vi "check noise source.vi"(8 "PLC bool write Tags":T1={"AT set glass wand lower"={"Tag Name"="S060.PXI.Signals.PlltData.SN", "Network Path"="172.15.51.1,1,0", "use opc"=FALSE, "DataSocket Reference"={"CWDSLib._DCWDataSocket"=refnum, "CWDSLib._DCWData"=refnum, "OnDataUpdated"=0, "OnStatusUpdated"=0}}, "AT set sunshade wand lower"={"Tag Name"="S060.PXI.Signals.PlltData.SN", "Network Path"="172.15.51.1,1,0", "use opc"=FALSE, "DataSocket Reference"={"CWDSLib._DCWDataSocket"=refnum, "CWDSLib._DCWData"=refnum, "OnDataUpdated"=0, "OnStatusUpdated"=0}}, "AT set sunshade wand up"={"Tag Name"="S060.PXI.Signals.PlltData.SN", "Network Path"="172.15.51.1,1,0", "use opc"=FALSE, "DataSocket Reference"={"CWDSLib._DCWDataSocket"=refnum, "CWDSLib._DCWData"=refnum, "OnDataUpdated"=0, "OnStatusUpdated"=0}}, "AT set glass wand up"={"Tag Name"="S060.PXI.Signals.PlltData.SN", "Network Path"="172.15.51.1,1,0", "use opc"=FALSE, "DataSocket Reference"={"CWDSLib._DCWDataSocket"=refnum, "CWDSLib._DCWData"=refnum, "OnDataUpdated"=0, "OnStatusUpdated"=0}}, "AT set wand home pos"={"Tag Name"="S060.PXI.Signals.PlltData.SN", "Network Path"="172.15.51.1,1,0", "use opc"=FALSE, "DataSocket Reference"={"CWDSLib._DCWDataSocket"=refnum, "CWDSLib._DCWData"=refnum, "OnDataUpdated"=0, "OnStatusUpdated"=0}}, "Test Complete Pass"={"Tag Name"="S060.PXI.Signals.PlltData.SN", "Network Path"="172.15.51.1,1,0", "use opc"=FALSE, "DataSocket Reference"={"CWDSLib._DCWDataSocket"=refnum, "CWDSLib._DCWData"=refnum, "OnDataUpdated"=0, "OnStatusUpdated"=0}}, "Test Complete Fail"={"Tag Name"="S060.PXI.Signals.PlltData.SN", "Network Path"="172.15.51.1,1,0", "use opc"=FALSE, "DataSocket Reference"={"CWDSLib._DCWDataSocket"=refnum, "CWDSLib._DCWData"=refnum, "OnDataUpdated"=0, "OnStatusUpdated"=0}}, "Test Started"={"Tag Name"="S060.PXI.Signals.PlltData.SN", "Network Path"="172.15.51.1,1,0", "use opc"=FALSE, "DataSocket Reference"={"CWDSLib._DCWDataSocket"=refnum, "CWDSLib._DCWData"=refnum, "OnDataUpdated"=0, "OnStatusUpdated"=0}}, "Retract LVDT's"={"Tag Name"="S060.PXI.Signals.PlltData.SN", "Network Path"="172.15.51.1,1,0", "use opc"=FALSE, "DataSocket Reference"={"CWDSLib._DCWDataSocket"=refnum, "CWDSLib._DCWData"=refnum, "OnDataUpdated"=0, "OnStatusUpdated"=0}}, "Extend LVDT's"={"Tag Name"="S060.PXI.Signals.PlltData.SN", "Network Path"="172.15.51.1,1,0", "use opc"=FALSE, "DataSocket Reference"={"CWDSLib._DCWDataSocket"=refnum, "CWDSLib._DCWData"=refnum, "OnDataUpdated"=0, "OnStatusUpdated"=0}}, "ss servo open"={"Tag Name"="S060.PXI.Signals.PlltData.SN", "Network Path"="172.15.51.1,1,0", "use opc"=FALSE, "DataSocket Reference"={"CWDSLib._DCWDataSocket"=refnum, "CWDSLib._DCWData"=refnum, "OnDataUpdated"=0, "OnStatusUpdated"=0}}, "ss servo close"={"Tag Name"="S060.PXI.Signals.PlltData.SN", "Network Path"="172.15.51.1,1,0", "use opc"=FALSE, "DataSocket Reference"={"CWDSLib._DCWDataSocket"=refnum, "CWDSLib._DCWData"=refnum, "OnDataUpdated"=0, "OnStatusUpdated"=0}}, "control slide start"={"Tag Name"="S060.PXI.Signals.PlltData.SN", "Network Path"="172.15.51.1,1,0", "use opc"=FALSE, "DataSocket Reference"={"CWDSLib._DCWDataSocket"=refnum, "CWDSLib._DCWData"=refnum, "OnDataUpdated"=0, "OnStatusUpdated"=0}}, "control slide stop"={"Tag Name"="S060.PXI.Signals.PlltData.SN", "Network Path"="172.15.51.1,1,0", "use opc"=FALSE, "DataSocket Reference"={"CWDSLib._DCWDataSocket"=refnum, "CWDSLib._DCWData"=refnum, "OnDataUpdated"=0, "OnStatusUpdated"=0}}, "AT VentPMACHome"={"Tag Name"="S060.PXI.Signals.PlltData.SN", "Network Path"="172.15.51.1,1,0", "use opc"=FALSE, "DataSocket Reference"={"CWDSLib._DCWDataSocket"=refnum, "CWDSLib._DCWData"=refnum, "OnDataUpdated"=0, "OnStatusUpdated"=0}}, "AT VentPMACExtended"={"Tag Name"="S060.PXI.Signals.PlltData.SN", "Network Path"="172.15.51.1,1,0", "use opc"=FALSE, "DataSocket Reference"={"CWDSLib._DCWDataSocket"=refnum, "CWDSLib._DCWData"=refnum, "OnDataUpdated"=0, "OnStatusUpdated"=0}}, "Good Frame Barcode"={"Tag Name"="S060.PXI.Signals.PlltData.SN", "Network Path"="172.15.51.1,1,0", "use opc"=FALSE, "DataSocket Reference"={"CWDSLib._DCWDataSocket"=refnum, "CWDSLib._DCWData"=refnum, "OnDataUpdated"=0, "OnStatusUpdated"=0}}, "Bad Frame Barcode"={"Tag Name"="S060.PXI.Signals.PlltData.SN", "Network Path"="172.15.51.1,1,0", "use opc"=FALSE, "DataSocket Reference"={"CWDSLib._DCWDataSocket"=refnum, "CWDSLib._DCWData"=refnum, "OnDataUpdated"=0, "OnStatusUpdated"=0}}, "Extend Z LVDTS"={"Tag Name"="S060.PXI.Signals.PlltData.SN", "Network Path"="172.15.51.1,1,0", "use opc"=FALSE, "DataSocket Reference"={"CWDSLib._DCWDataSocket"=refnum, "CWDSLib._DCWData"=refnum, "OnDataUpdated"=0, "OnStatusUpdated"=0}}, "NVH SunRoof Moving"={"Tag Name"="S060.PXI.Signals.PlltData.SN", "Network Path"="172.15.51.1,1,0", "use opc"=FALSE, "DataSocket Reference"={"CWDSLib._DCWDataSocket"=refnum, "CWDSLib._DCWData"=refnum, "OnDataUpdated"=0, "OnStatusUpdated"=0}}, "NVH SunRoof Stop"={"Tag Name"="S060.PXI.Signals.PlltData.SN", "Network Path"="172.15.51.1,1,0", "use opc"=FALSE, "DataSocket Reference"={"CWDSLib._DCWDataSocket"=refnum, "CWDSLib._DCWData"=refnum, "OnDataUpdated"=0, "OnStatusUpdated"=0}}, "NVH Pass"={"Tag Name"="S060.PXI.Signals.PlltData.SN", "Network Path"="172.15.51.1,1,0", "use opc"=FALSE, "DataSocket Reference"={"CWDSLib._DCWDataSocket"=refnum, "CWDSLib._DCWData"=refnum, "OnDataUpdated"=0, "OnStatusUpdated"=0}}, "NVH Fail"={"Tag Name"="S060.PXI.Signals.PlltData.SN", "Network Path"="172.15.51.1,1,0", "use opc"=FALSE, "DataSocket Reference"={"CWDSLib._DCWDataSocket"=refnum, "CWDSLib._DCWData"=refnum, "OnDataUpdated"=0, "OnStatusUpdated"=0}}, "NVH Operator Express Glass Opened"={"Tag Name"="S060.PXI.Signals.PlltData.SN", "Network Path"="172.15.51.1,1,0", "use opc"=FALSE, "DataSocket Reference"={"CWDSLib._DCWDataSocket"=refnum, "CWDSLib._DCWData"=refnum, "OnDataUpdated"=0, "OnStatusUpdated"=0}}, "NVH Operator Express Glass Closed"={"Tag Name"="S060.PXI.Signals.PlltData.SN", "Network Path"="172.15.51.1,1,0", "use opc"=FALSE, "DataSocket Reference"={"CWDSLib._DCWDataSocket"=refnum, "CWDSLib._DCWData"=refnum, "OnDataUpdated"=0, "OnStatusUpdated"=0}}, "NVH Operator Express Rollo Opened01"={"Tag Name"="S060.PXI.Signals.PlltData.SN", "Network Path"="172.15.51.1,1,0", "use opc"=FALSE, "DataSocket Reference"={"CWDSLib._DCWDataSocket"=refnum, "CWDSLib._DCWData"=refnum, "OnDataUpdated"=0, "OnStatusUpdated"=0}}, "NVH Operator Express Rollo Closed01"={"Tag Name"="S060.PXI.Signals.PlltData.SN", "Network Path"="172.15.51.1,1,0", "use opc"=FALSE, "DataSocket Reference"={"CWDSLib._DCWDataSocket"=refnum, "CWDSLib._DCWData"=refnum, "OnDataUpdated"=0, "OnStatusUpdated"=0}}, "NVH Operator Express Rollo Opened02"={"Tag Name"="S060.PXI.Signals.PlltData.SN", "Network Path"="172.15.51.1,1,0", "use opc"=FALSE, "DataSocket Reference"={"CWDSLib._DCWDataSocket"=refnum, "CWDSLib._DCWData"=refnum, "OnDataUpdated"=0, "OnStatusUpdated"=0}}, "NVH Operator Pass"={"Tag Name"="S060.PXI.Signals.PlltData.SN", "Network Path"="172.15.51.1,1,0", "use opc"=FALSE, "DataSocket Reference"={"CWDSLib._DCWDataSocket"=refnum, "CWDSLib._DCWData"=refnum, "OnDataUpdated"=0, "OnStatusUpdated"=0}}, "NVH Operator Fail"={"Tag Name"="S060.PXI.Signals.PlltData.SN", "Network Path"="172.15.51.1,1,0", "use opc"=FALSE, "DataSocket Reference"={"CWDSLib._DCWDataSocket"=refnum, "CWDSLib._DCWData"=refnum, "OnDataUpdated"=0, "OnStatusUpdated"=0}}, "NVH Operator Check"={"Tag Name"="S060.PXI.Signals.PlltData.SN", "Network Path"="172.15.51.1,1,0", "use opc"=FALSE, "DataSocket Reference"={"CWDSLib._DCWDataSocket"=refnum, "CWDSLib._DCWData"=refnum, "OnDataUpdated"=0, "OnStatusUpdated"=0}}, "NVH Operator Vent Open Noise"={"Tag Name"="S060.PXI.Signals.PlltData.SN", "Network Path"="172.15.51.1,1,0", "use opc"=FALSE, "DataSocket Reference"={"CWDSLib._DCWDataSocket"=refnum, "CWDSLib._DCWData"=refnum, "OnDataUpdated"=0, "OnStatusUpdated"=0}}, "NVH Operator Vent Close Noise"={"Tag Name"="S060.PXI.Signals.PlltData.SN", "Network Path"="172.15.51.1,1,0", "use opc"=FALSE, "DataSocket Reference"={"CWDSLib._DCWDataSocket"=refnum, "CWDSLib._DCWData"=refnum, "OnDataUpdated"=0, "OnStatusUpdated"=0}}, "NVH Operator Sunshade Open Noise"={"Tag Name"="S060.PXI.Signals.PlltData.SN", "Network Path"="172.15.51.1,1,0", "use opc"=FALSE, "DataSocket Reference"={"CWDSLib._DCWDataSocket"=refnum, "CWDSLib._DCWData"=refnum, "OnDataUpdated"=0, "OnStatusUpdated"=0}}, "NVH Operator Sunshade Close Noise"={"Tag Name"="S060.PXI.Signals.PlltData.SN", "Network Path"="172.15.51.1,1,0", "use opc"=FALSE, "DataSocket Reference"={"CWDSLib._DCWDataSocket"=refnum, "CWDSLib._DCWData"=refnum, "OnDataUpdated"=0, "OnStatusUpdated"=0}}, "NVH Operator Glass Open Noise"={"Tag Name"="S060.PXI.Signals.PlltData.SN", "Network Path"="172.15.51.1,1,0", "use opc"=FALSE, "DataSocket Reference"={"CWDSLib._DCWDataSocket"=refnum, "CWDSLib._DCWData"=refnum, "OnDataUpdated"=0, "OnStatusUpdated"=0}}, "NVH Operator Glass Close Noise"={"Tag Name"="S060.PXI.Signals.PlltData.SN", "Network Path"="172.15.51.1,1,0", "use opc"=FALSE, "DataSocket Reference"={"CWDSLib._DCWDataSocket"=refnum, "CWDSLib._DCWData"=refnum, "OnDataUpdated"=0, "OnStatusUpdated"=0}}, "NVH Operator Finish"={"Tag Name"="S060.PXI.Signals.PlltData.SN", "Network Path"="172.15.51.1,1,0", "use opc"=FALSE, "DataSocket Reference"={"CWDSLib._DCWDataSocket"=refnum, "CWDSLib._DCWData"=refnum, "OnDataUpdated"=0, "OnStatusUpdated"=0}}, "Barcode01 OK"={"Tag Name"="S060.PXI.Signals.PlltData.SN", "Network Path"="172.15.51.1,1,0", "use opc"=FALSE, "DataSocket Reference"={"CWDSLib._DCWDataSocket"=refnum, "CWDSLib._DCWData"=refnum, "OnDataUpdated"=0, "OnStatusUpdated"=0}}, "Barcode02 OK"={"Tag Name"="S060.PXI.Signals.PlltData.SN", "Network Path"="172.15.51.1,1,0", "use opc"=FALSE, "DataSocket Reference"={"CWDSLib._DCWDataSocket"=refnum, "CWDSLib._DCWData"=refnum, "OnDataUpdated"=0, "OnStatusUpdated"=0}}, "AT set to Vent ATS Test Pos"={"Tag Name"="S060.PXI.Signals.PlltData.SN", "Network Path"="172.15.51.1,1,0", "use opc"=FALSE, "DataSocket Reference"={"CWDSLib._DCWDataSocket"=refnum, "CWDSLib._DCWData"=refnum, "OnDataUpdated"=0, "OnStatusUpdated"=0}}, "AT set to Vent ATS Home Pos"={"Tag Name"="S060.PXI.Signals.PlltData.SN", "Network Path"="172.15.51.1,1,0", "use opc"=FALSE, "DataSocket Reference"={"CWDSLib._DCWDataSocket"=refnum, "CWDSLib._DCWData"=refnum, "OnDataUpdated"=0, "OnStatusUpdated"=0}}, "Move LVDT Adjust Station"={"Tag Name"="S060.PXI.Signals.PlltData.SN", "Network Path"="172.15.51.1,1,0", "use opc"=FALSE, "DataSocket Reference"={"CWDSLib._DCWDataSocket"=refnum, "CWDSLib._DCWData"=refnum, "OnDataUpdated"=0, "OnStatusUpdated"=0}}} {"Move LVDT Adjust Station"."DataSocket Reference"."OnStatusUpdated" format="%.0x"; "Move LVDT Adjust Station"."DataSocket Reference"."OnDataUpdated" format="%.0x"; "AT set to Vent ATS Home Pos"."DataSocket Reference"."OnStatusUpdated" format="%.0x"; "AT set to Vent ATS Home Pos"."DataSocket Reference"."OnDataUpdated" format="%.0x"; "AT set to Vent ATS Test Pos"."DataSocket Reference"."OnStatusUpdated" format="%.0x"; "AT set to Vent ATS Test Pos"."DataSocket Reference"."OnDataUpdated" format="%.0x"; "Barcode02 OK"."DataSocket Reference"."OnStatusUpdated" format="%.0x"; "Barcode02 OK"."DataSocket Reference"."OnDataUpdated" format="%.0x"; "Barcode01 OK"."DataSocket Reference"."OnStatusUpdated" format="%.0x"; "Barcode01 OK"."DataSocket Reference"."OnDataUpdated" format="%.0x"; "AT set glass wand up"."DataSocket Reference"."OnStatusUpdated" format="%.0x"; "AT set glass wand up"."DataSocket Reference"."OnDataUpdated" format="%.0x"; "AT set sunshade wand up"."DataSocket Reference"."OnStatusUpdated" format="%.0x"; "AT set sunshade wand up"."DataSocket Reference"."OnDataUpdated" format="%.0x"; "NVH Operator Finish"."DataSocket Reference"."OnStatusUpdated" format="%.0x"; "NVH Operator Finish"."DataSocket Reference"."OnDataUpdated" format="%.0x"; "NVH Operator Glass Close Noise"."DataSocket Reference"."OnStatusUpdated" format="%.0x"; "NVH Operator Glass Close Noise"."DataSocket Reference"."OnDataUpdated" format="%.0x"; "NVH Operator Glass Open Noise"."DataSocket Reference"."OnStatusUpdated" format="%.0x"; "NVH Operator Glass Open Noise"."DataSocket Reference"."OnDataUpdated" format="%.0x"; "NVH Operator Sunshade Close Noise"."DataSocket Reference"."OnStatusUpdated" format="%.0x"; "NVH Operator Sunshade Close Noise"."DataSocket Reference"."OnDataUpdated" format="%.0x"; "NVH Operator Sunshade Open Noise"."DataSocket Reference"."OnStatusUpdated" format="%.0x"; "NVH Operator Sunshade Open Noise"."DataSocket Reference"."OnDataUpdated" format="%.0x"; "NVH Operator Vent Close Noise"."DataSocket Reference"."OnStatusUpdated" format="%.0x"; "NVH Operator Vent Close Noise"."DataSocket Reference"."OnDataUpdated" format="%.0x"; "NVH Operator Vent Open Noise"."DataSocket Reference"."OnStatusUpdated" format="%.0x"; "NVH Operator Vent Open Noise"."DataSocket Reference"."OnDataUpdated" format="%.0x"; "NVH Operator Check"."DataSocket Reference"."OnStatusUpdated" format="%.0x"; "NVH Operator Check"."DataSocket Reference"."OnDataUpdated" format="%.0x"; "NVH Operator Fail"."DataSocket Reference"."OnStatusUpdated" format="%.0x"; "NVH Operator Fail"."DataSocket Reference"."OnDataUpdated" format="%.0x"; "NVH Operator Pass"."DataSocket Reference"."OnStatusUpdated" format="%.0x"; "NVH Operator Pass"."DataSocket Reference"."OnDataUpdated" format="%.0x"; "NVH Operator Express Rollo Opened02"."DataSocket Reference"."OnStatusUpdated" format="%.0x"; "NVH Operator Express Rollo Opened02"."DataSocket Reference"."OnDataUpdated" format="%.0x"; "NVH Operator Express Rollo Closed01"."DataSocket Reference"."OnStatusUpdated" format="%.0x"; "NVH Operator Express Rollo Closed01"."DataSocket Reference"."OnDataUpdated" format="%.0x"; "NVH Operator Express Rollo Opened01"."DataSocket Reference"."OnStatusUpdated" format="%.0x"; "NVH Operator Express Rollo Opened01"."DataSocket Reference"."OnDataUpdated" format="%.0x"; "NVH Operator Express Glass Closed"."DataSocket Reference"."OnStatusUpdated" format="%.0x"; "NVH Operator Express Glass Closed"."DataSocket Reference"."OnDataUpdated" format="%.0x"; "NVH Operator Express Glass Opened"."DataSocket Reference"."OnStatusUpdated" format="%.0x"; "NVH Operator Express Glass Opened"."DataSocket Reference"."OnDataUpdated" format="%.0x"; "NVH Fail"."DataSocket Reference"."OnStatusUpdated" format="%.0x"; "NVH Fail"."DataSocket Reference"."OnDataUpdated" format="%.0x"; "NVH Pass"."DataSocket Reference"."OnStatusUpdated" format="%.0x"; "NVH Pass"."DataSocket Reference"."OnDataUpdated" format="%.0x"; "NVH SunRoof Stop"."DataSocket Reference"."OnStatusUpdated" format="%.0x"; "NVH SunRoof Stop"."DataSocket Reference"."OnDataUpdated" format="%.0x"; "NVH SunRoof Moving"."DataSocket Reference"."OnStatusUpdated" format="%.0x"; "NVH SunRoof Moving"."DataSocket Reference"."OnDataUpdated" format="%.0x"; "Extend Z LVDTS"."DataSocket Reference"."OnStatusUpdated" format="%.0x"; "Extend Z LVDTS"."DataSocket Reference"."OnDataUpdated" format="%.0x"; "Bad Frame Barcode"."DataSocket Reference"."OnStatusUpdated" format="%.0x"; "Bad Frame Barcode"."DataSocket Reference"."OnDataUpdated" format="%.0x"; "Good Frame Barcode"."DataSocket Reference"."OnStatusUpdated" format="%.0x"; "Good Frame Barcode"."DataSocket Reference"."OnDataUpdated" format="%.0x"; "AT VentPMACExtended"."DataSocket Reference"."OnStatusUpdated" format="%.0x"; "AT VentPMACExtended"."DataSocket Reference"."OnDataUpdated" format="%.0x"; "AT VentPMACHome"."DataSocket Reference"."OnStatusUpdated" format="%.0x"; "AT VentPMACHome"."DataSocket Reference"."OnDataUpdated" format="%.0x"; "control slide stop"."DataSocket Reference"."OnStatusUpdated" format="%.0x"; "control slide stop"."DataSocket Reference"."OnDataUpdated" format="%.0x"; "control slide start"."DataSocket Reference"."OnStatusUpdated" format="%.0x"; "control slide start"."DataSocket Reference"."OnDataUpdated" format="%.0x"; "ss servo close"."DataSocket Reference"."OnStatusUpdated" format="%.0x"; "ss servo close"."DataSocket Reference"."OnDataUpdated" format="%.0x"; "ss servo open"."DataSocket Reference"."OnStatusUpdated" format="%.0x"; "ss servo open"."DataSocket Reference"."OnDataUpdated" format="%.0x"; "Extend LVDT's"."DataSocket Reference"."OnStatusUpdated" format="%.0x"; "Extend LVDT's"."DataSocket Reference"."OnDataUpdated" format="%.0x"; "Retract LVDT's"."DataSocket Reference"."OnStatusUpdated" format="%.0x"; "Retract LVDT's"."DataSocket Reference"."OnDataUpdated" format="%.0x"; "Test Started"."DataSocket Reference"."OnStatusUpdated" format="%.0x"; "Test Started"."DataSocket Reference"."OnDataUpdated" format="%.0x"; "Test Complete Fail"."DataSocket Reference"."OnStatusUpdated" format="%.0x"; "Test Complete Fail"."DataSocket Reference"."OnDataUpdated" format="%.0x"; "Test Complete Pass"."DataSocket Reference"."OnStatusUpdated" format="%.0x"; "Test Complete Pass"."DataSocket Reference"."OnDataUpdated" format="%.0x"; "AT set wand home pos"."DataSocket Reference"."OnStatusUpdated" format="%.0x"; "AT set wand home pos"."DataSocket Reference"."OnDataUpdated" format="%.0x"; "AT set sunshade wand lower"."DataSocket Reference"."OnStatusUpdated" format="%.0x"; "AT set sunshade wand lower"."DataSocket Reference"."OnDataUpdated" format="%.0x"; "AT set glass wand lower"."DataSocket Reference"."OnStatusUpdated" format="%.0x"; "AT set glass wand lower"."DataSocket Reference"."OnDataUpdated" format="%.0x"}, 9 "Noise Source Input":u32, 10 "Error Table In":string[][](table), 11 "input cluster":T4={"AT glass position"={"Tag Name"="S060.PXI.Signals.PlltData.SN", "Network Path"="172.15.51.1,1,0", "use opc"=FALSE, "DataSocket Reference"={"CWDSLib._DCWDataSocket"=refnum, "CWDSLib._DCWData"=refnum, "OnDataUpdated"=0, "OnStatusUpdated"=0}}, "AT shade position"={"Tag Name"="S060.PXI.Signals.PlltData.SN", "Network Path"="172.15.51.1,1,0", "use opc"=FALSE, "DataSocket Reference"={"CWDSLib._DCWDataSocket"=refnum, "CWDSLib._DCWData"=refnum, "OnDataUpdated"=0, "OnStatusUpdated"=0}}, "AT in glass wand lower pos"={"Tag Name"="S060.PXI.Signals.PlltData.SN", "Network Path"="172.15.51.1,1,0", "use opc"=FALSE, "DataSocket Reference"={"CWDSLib._DCWDataSocket"=refnum, "CWDSLib._DCWData"=refnum, "OnDataUpdated"=0, "OnStatusUpdated"=0}}, "AT in glass wand up pos"={"Tag Name"="S060.PXI.Signals.PlltData.SN", "Network Path"="172.15.51.1,1,0", "use opc"=FALSE, "DataSocket Reference"={"CWDSLib._DCWDataSocket"=refnum, "CWDSLib._DCWData"=refnum, "OnDataUpdated"=0, "OnStatusUpdated"=0}}, "AT in sunshad wand lower pos"={"Tag Name"="S060.PXI.Signals.PlltData.SN", "Network Path"="172.15.51.1,1,0", "use opc"=FALSE, "DataSocket Reference"={"CWDSLib._DCWDataSocket"=refnum, "CWDSLib._DCWData"=refnum, "OnDataUpdated"=0, "OnStatusUpdated"=0}}, "AT in sunshad wand up pos"={"Tag Name"="S060.PXI.Signals.PlltData.SN", "Network Path"="172.15.51.1,1,0", "use opc"=FALSE, "DataSocket Reference"={"CWDSLib._DCWDataSocket"=refnum, "CWDSLib._DCWData"=refnum, "OnDataUpdated"=0, "OnStatusUpdated"=0}}, "AT in wand home pos"={"Tag Name"="S060.PXI.Signals.PlltData.SN", "Network Path"="172.15.51.1,1,0", "use opc"=FALSE, "DataSocket Reference"={"CWDSLib._DCWDataSocket"=refnum, "CWDSLib._DCWData"=refnum, "OnDataUpdated"=0, "OnStatusUpdated"=0}}, "LVDT's Extended"={"Tag Name"="S060.PXI.Signals.PlltData.SN", "Network Path"="172.15.51.1,1,0", "use opc"=FALSE, "DataSocket Reference"={"CWDSLib._DCWDataSocket"=refnum, "CWDSLib._DCWData"=refnum, "OnDataUpdated"=0, "OnStatusUpdated"=0}}, "bolt check 1"={"Tag Name"="S060.PXI.Signals.PlltData.SN", "Network Path"="172.15.51.1,1,0", "use opc"=FALSE, "DataSocket Reference"={"CWDSLib._DCWDataSocket"=refnum, "CWDSLib._DCWData"=refnum, "OnDataUpdated"=0, "OnStatusUpdated"=0}}, "bolt check 2"={"Tag Name"="S060.PXI.Signals.PlltData.SN", "Network Path"="172.15.51.1,1,0", "use opc"=FALSE, "DataSocket Reference"={"CWDSLib._DCWDataSocket"=refnum, "CWDSLib._DCWData"=refnum, "OnDataUpdated"=0, "OnStatusUpdated"=0}}, "bolt check 3"={"Tag Name"="S060.PXI.Signals.PlltData.SN", "Network Path"="172.15.51.1,1,0", "use opc"=FALSE, "DataSocket Reference"={"CWDSLib._DCWDataSocket"=refnum, "CWDSLib._DCWData"=refnum, "OnDataUpdated"=0, "OnStatusUpdated"=0}}, "bolt check 4"={"Tag Name"="S060.PXI.Signals.PlltData.SN", "Network Path"="172.15.51.1,1,0", "use opc"=FALSE, "DataSocket Reference"={"CWDSLib._DCWDataSocket"=refnum, "CWDSLib._DCWData"=refnum, "OnDataUpdated"=0, "OnStatusUpdated"=0}}, "bolt check 5"={"Tag Name"="S060.PXI.Signals.PlltData.SN", "Network Path"="172.15.51.1,1,0", "use opc"=FALSE, "DataSocket Reference"={"CWDSLib._DCWDataSocket"=refnum, "CWDSLib._DCWData"=refnum, "OnDataUpdated"=0, "OnStatusUpdated"=0}}, "bolt check 6"={"Tag Name"="S060.PXI.Signals.PlltData.SN", "Network Path"="172.15.51.1,1,0", "use opc"=FALSE, "DataSocket Reference"={"CWDSLib._DCWDataSocket"=refnum, "CWDSLib._DCWData"=refnum, "OnDataUpdated"=0, "OnStatusUpdated"=0}}, "bolt check 7"={"Tag Name"="S060.PXI.Signals.PlltData.SN", "Network Path"="172.15.51.1,1,0", "use opc"=FALSE, "DataSocket Reference"={"CWDSLib._DCWDataSocket"=refnum, "CWDSLib._DCWData"=refnum, "OnDataUpdated"=0, "OnStatusUpdated"=0}}, "bolt check 8"={"Tag Name"="S060.PXI.Signals.PlltData.SN", "Network Path"="172.15.51.1,1,0", "use opc"=FALSE, "DataSocket Reference"={"CWDSLib._DCWDataSocket"=refnum, "CWDSLib._DCWData"=refnum, "OnDataUpdated"=0, "OnStatusUpdated"=0}}, "start"={"Tag Name"="S060.PXI.Signals.PlltData.SN", "Network Path"="172.15.51.1,1,0", "use opc"=FALSE, "DataSocket Reference"={"CWDSLib._DCWDataSocket"=refnum, "CWDSLib._DCWData"=refnum, "OnDataUpdated"=0, "OnStatusUpdated"=0}}, "abort"={"Tag Name"="S060.PXI.Signals.PlltData.SN", "Network Path"="172.15.51.1,1,0", "use opc"=FALSE, "DataSocket Reference"={"CWDSLib._DCWDataSocket"=refnum, "CWDSLib._DCWData"=refnum, "OnDataUpdated"=0, "OnStatusUpdated"=0}}, "LVDT's Retracted"={"Tag Name"="S060.PXI.Signals.PlltData.SN", "Network Path"="172.15.51.1,1,0", "use opc"=FALSE, "DataSocket Reference"={"CWDSLib._DCWDataSocket"=refnum, "CWDSLib._DCWData"=refnum, "OnDataUpdated"=0, "OnStatusUpdated"=0}}, "manual barcode print"={"Tag Name"="S060.PXI.Signals.PlltData.SN", "Network Path"="172.15.51.1,1,0", "use opc"=FALSE, "DataSocket Reference"={"CWDSLib._DCWDataSocket"=refnum, "CWDSLib._DCWData"=refnum, "OnDataUpdated"=0, "OnStatusUpdated"=0}}, "ss servo at open"={"Tag Name"="S060.PXI.Signals.PlltData.SN", "Network Path"="172.15.51.1,1,0", "use opc"=FALSE, "DataSocket Reference"={"CWDSLib._DCWDataSocket"=refnum, "CWDSLib._DCWData"=refnum, "OnDataUpdated"=0, "OnStatusUpdated"=0}}, "ss servo at close"={"Tag Name"="S060.PXI.Signals.PlltData.SN", "Network Path"="172.15.51.1,1,0", "use opc"=FALSE, "DataSocket Reference"={"CWDSLib._DCWDataSocket"=refnum, "CWDSLib._DCWData"=refnum, "OnDataUpdated"=0, "OnStatusUpdated"=0}}, "ss servo opening"={"Tag Name"="S060.PXI.Signals.PlltData.SN", "Network Path"="172.15.51.1,1,0", "use opc"=FALSE, "DataSocket Reference"={"CWDSLib._DCWDataSocket"=refnum, "CWDSLib._DCWData"=refnum, "OnDataUpdated"=0, "OnStatusUpdated"=0}}, "ss servo closing"={"Tag Name"="S060.PXI.Signals.PlltData.SN", "Network Path"="172.15.51.1,1,0", "use opc"=FALSE, "DataSocket Reference"={"CWDSLib._DCWDataSocket"=refnum, "CWDSLib._DCWData"=refnum, "OnDataUpdated"=0, "OnStatusUpdated"=0}}, "control slide at home"={"Tag Name"="S060.PXI.Signals.PlltData.SN", "Network Path"="172.15.51.1,1,0", "use opc"=FALSE, "DataSocket Reference"={"CWDSLib._DCWDataSocket"=refnum, "CWDSLib._DCWData"=refnum, "OnDataUpdated"=0, "OnStatusUpdated"=0}}, "control slide left good"={"Tag Name"="S060.PXI.Signals.PlltData.SN", "Network Path"="172.15.51.1,1,0", "use opc"=FALSE, "DataSocket Reference"={"CWDSLib._DCWDataSocket"=refnum, "CWDSLib._DCWData"=refnum, "OnDataUpdated"=0, "OnStatusUpdated"=0}}, "control slide left over stroke"={"Tag Name"="S060.PXI.Signals.PlltData.SN", "Network Path"="172.15.51.1,1,0", "use opc"=FALSE, "DataSocket Reference"={"CWDSLib._DCWDataSocket"=refnum, "CWDSLib._DCWData"=refnum, "OnDataUpdated"=0, "OnStatusUpdated"=0}}, "control slide right good"={"Tag Name"="S060.PXI.Signals.PlltData.SN", "Network Path"="172.15.51.1,1,0", "use opc"=FALSE, "DataSocket Reference"={"CWDSLib._DCWDataSocket"=refnum, "CWDSLib._DCWData"=refnum, "OnDataUpdated"=0, "OnStatusUpdated"=0}}, "control slide right over stroke"={"Tag Name"="S060.PXI.Signals.PlltData.SN", "Network Path"="172.15.51.1,1,0", "use opc"=FALSE, "DataSocket Reference"={"CWDSLib._DCWDataSocket"=refnum, "CWDSLib._DCWData"=refnum, "OnDataUpdated"=0, "OnStatusUpdated"=0}}, "wind deflector high speed pos"={"Tag Name"="S060.PXI.Signals.PlltData.SN", "Network Path"="172.15.51.1,1,0", "use opc"=FALSE, "DataSocket Reference"={"CWDSLib._DCWDataSocket"=refnum, "CWDSLib._DCWData"=refnum, "OnDataUpdated"=0, "OnStatusUpdated"=0}}, "wind deflector low speed pos"={"Tag Name"="S060.PXI.Signals.PlltData.SN", "Network Path"="172.15.51.1,1,0", "use opc"=FALSE, "DataSocket Reference"={"CWDSLib._DCWDataSocket"=refnum, "CWDSLib._DCWData"=refnum, "OnDataUpdated"=0, "OnStatusUpdated"=0}}, "AT VentPMACatHome"={"Tag Name"="S060.PXI.Signals.PlltData.SN", "Network Path"="172.15.51.1,1,0", "use opc"=FALSE, "DataSocket Reference"={"CWDSLib._DCWDataSocket"=refnum, "CWDSLib._DCWData"=refnum, "OnDataUpdated"=0, "OnStatusUpdated"=0}}, "AT VentPMACisExtend"={"Tag Name"="S060.PXI.Signals.PlltData.SN", "Network Path"="172.15.51.1,1,0", "use opc"=FALSE, "DataSocket Reference"={"CWDSLib._DCWDataSocket"=refnum, "CWDSLib._DCWData"=refnum, "OnDataUpdated"=0, "OnStatusUpdated"=0}}, "SS Barcode Scanner Bypassed"={"Tag Name"="S060.PXI.Signals.PlltData.SN", "Network Path"="172.15.51.1,1,0", "use opc"=FALSE, "DataSocket Reference"={"CWDSLib._DCWDataSocket"=refnum, "CWDSLib._DCWData"=refnum, "OnDataUpdated"=0, "OnStatusUpdated"=0}}, "Check Frame Barcode"={"Tag Name"="S060.PXI.Signals.PlltData.SN", "Network Path"="172.15.51.1,1,0", "use opc"=FALSE, "DataSocket Reference"={"CWDSLib._DCWDataSocket"=refnum, "CWDSLib._DCWData"=refnum, "OnDataUpdated"=0, "OnStatusUpdated"=0}}, "Z LVDTs Extended"={"Tag Name"="S060.PXI.Signals.PlltData.SN", "Network Path"="172.15.51.1,1,0", "use opc"=FALSE, "DataSocket Reference"={"CWDSLib._DCWDataSocket"=refnum, "CWDSLib._DCWData"=refnum, "OnDataUpdated"=0, "OnStatusUpdated"=0}}, "NVH Operator Pass"={"Tag Name"="S060.PXI.Signals.PlltData.SN", "Network Path"="172.15.51.1,1,0", "use opc"=FALSE, "DataSocket Reference"={"CWDSLib._DCWDataSocket"=refnum, "CWDSLib._DCWData"=refnum, "OnDataUpdated"=0, "OnStatusUpdated"=0}}, "NVH Operator Fail"={"Tag Name"="S060.PXI.Signals.PlltData.SN", "Network Path"="172.15.51.1,1,0", "use opc"=FALSE, "DataSocket Reference"={"CWDSLib._DCWDataSocket"=refnum, "CWDSLib._DCWData"=refnum, "OnDataUpdated"=0, "OnStatusUpdated"=0}}, "NVH Operator Express Glass Open"={"Tag Name"="S060.PXI.Signals.PlltData.SN", "Network Path"="172.15.51.1,1,0", "use opc"=FALSE, "DataSocket Reference"={"CWDSLib._DCWDataSocket"=refnum, "CWDSLib._DCWData"=refnum, "OnDataUpdated"=0, "OnStatusUpdated"=0}}, "NVH Operator Express Glass Close"={"Tag Name"="S060.PXI.Signals.PlltData.SN", "Network Path"="172.15.51.1,1,0", "use opc"=FALSE, "DataSocket Reference"={"CWDSLib._DCWDataSocket"=refnum, "CWDSLib._DCWData"=refnum, "OnDataUpdated"=0, "OnStatusUpdated"=0}}, "NVH Operator Express Rollo Open01"={"Tag Name"="S060.PXI.Signals.PlltData.SN", "Network Path"="172.15.51.1,1,0", "use opc"=FALSE, "DataSocket Reference"={"CWDSLib._DCWDataSocket"=refnum, "CWDSLib._DCWData"=refnum, "OnDataUpdated"=0, "OnStatusUpdated"=0}}, "NVH Operator Express Rollo Close01"={"Tag Name"="S060.PXI.Signals.PlltData.SN", "Network Path"="172.15.51.1,1,0", "use opc"=FALSE, "DataSocket Reference"={"CWDSLib._DCWDataSocket"=refnum, "CWDSLib._DCWData"=refnum, "OnDataUpdated"=0, "OnStatusUpdated"=0}}, "NVH Operator Express Rollo Open02"={"Tag Name"="S060.PXI.Signals.PlltData.SN", "Network Path"="172.15.51.1,1,0", "use opc"=FALSE, "DataSocket Reference"={"CWDSLib._DCWDataSocket"=refnum, "CWDSLib._DCWData"=refnum, "OnDataUpdated"=0, "OnStatusUpdated"=0}}, "NVH Operator Express Rollo Close02"={"Tag Name"="S060.PXI.Signals.PlltData.SN", "Network Path"="172.15.51.1,1,0", "use opc"=FALSE, "DataSocket Reference"={"CWDSLib._DCWDataSocket"=refnum, "CWDSLib._DCWData"=refnum, "OnDataUpdated"=0, "OnStatusUpdated"=0}}, "NVH Operator Vent Open Noise"={"Tag Name"="S060.PXI.Signals.PlltData.SN", "Network Path"="172.15.51.1,1,0", "use opc"=FALSE, "DataSocket Reference"={"CWDSLib._DCWDataSocket"=refnum, "CWDSLib._DCWData"=refnum, "OnDataUpdated"=0, "OnStatusUpdated"=0}}, "NVH Operator Vent Close Noise"={"Tag Name"="S060.PXI.Signals.PlltData.SN", "Network Path"="172.15.51.1,1,0", "use opc"=FALSE, "DataSocket Reference"={"CWDSLib._DCWDataSocket"=refnum, "CWDSLib._DCWData"=refnum, "OnDataUpdated"=0, "OnStatusUpdated"=0}}, "NVH Operator Sunshade Open Noise"={"Tag Name"="S060.PXI.Signals.PlltData.SN", "Network Path"="172.15.51.1,1,0", "use opc"=FALSE, "DataSocket Reference"={"CWDSLib._DCWDataSocket"=refnum, "CWDSLib._DCWData"=refnum, "OnDataUpdated"=0, "OnStatusUpdated"=0}}, "NVH Operator Sunshade Close Noise"={"Tag Name"="S060.PXI.Signals.PlltData.SN", "Network Path"="172.15.51.1,1,0", "use opc"=FALSE, "DataSocket Reference"={"CWDSLib._DCWDataSocket"=refnum, "CWDSLib._DCWData"=refnum, "OnDataUpdated"=0, "OnStatusUpdated"=0}}, "NVH Operator Glass Open Noise"={"Tag Name"="S060.PXI.Signals.PlltData.SN", "Network Path"="172.15.51.1,1,0", "use opc"=FALSE, "DataSocket Reference"={"CWDSLib._DCWDataSocket"=refnum, "CWDSLib._DCWData"=refnum, "OnDataUpdated"=0, "OnStatusUpdated"=0}}, "NVH Operator Glass Close Noise"={"Tag Name"="S060.PXI.Signals.PlltData.SN", "Network Path"="172.15.51.1,1,0", "use opc"=FALSE, "DataSocket Reference"={"CWDSLib._DCWDataSocket"=refnum, "CWDSLib._DCWData"=refnum, "OnDataUpdated"=0, "OnStatusUpdated"=0}}, "NVH Operator Finish"={"Tag Name"="S060.PXI.Signals.PlltData.SN", "Network Path"="172.15.51.1,1,0", "use opc"=FALSE, "DataSocket Reference"={"CWDSLib._DCWDataSocket"=refnum, "CWDSLib._DCWData"=refnum, "OnDataUpdated"=0, "OnStatusUpdated"=0}}, "NVH Operator Check"={"Tag Name"="S060.PXI.Signals.PlltData.SN", "Network Path"="172.15.51.1,1,0", "use opc"=FALSE, "DataSocket Reference"={"CWDSLib._DCWDataSocket"=refnum, "CWDSLib._DCWData"=refnum, "OnDataUpdated"=0, "OnStatusUpdated"=0}}, "windproof position"={"Tag Name"="S060.PXI.Signals.PlltData.SN", "Network Path"="172.15.51.1,1,0", "use opc"=FALSE, "DataSocket Reference"={"CWDSLib._DCWDataSocket"=refnum, "CWDSLib._DCWData"=refnum, "OnDataUpdated"=0, "OnStatusUpdated"=0}}, "NVH Operator Express Glass vent Open"={"Tag Name"="S060.PXI.Signals.PlltData.SN", "Network Path"="172.15.51.1,1,0", "use opc"=FALSE, "DataSocket Reference"={"CWDSLib._DCWDataSocket"=refnum, "CWDSLib._DCWData"=refnum, "OnDataUpdated"=0, "OnStatusUpdated"=0}}, "NVH Operator Express Glass Vent Close"={"Tag Name"="S060.PXI.Signals.PlltData.SN", "Network Path"="172.15.51.1,1,0", "use opc"=FALSE, "DataSocket Reference"={"CWDSLib._DCWDataSocket"=refnum, "CWDSLib._DCWData"=refnum, "OnDataUpdated"=0, "OnStatusUpdated"=0}}, "NVH Operator Re-do"={"Tag Name"="S060.PXI.Signals.PlltData.SN", "Network Path"="172.15.51.1,1,0", "use opc"=FALSE, "DataSocket Reference"={"CWDSLib._DCWDataSocket"=refnum, "CWDSLib._DCWData"=refnum, "OnDataUpdated"=0, "OnStatusUpdated"=0}}, "AT at vent ATS test pos"={"Tag Name"="S060.PXI.Signals.PlltData.SN", "Network Path"="172.15.51.1,1,0", "use opc"=FALSE, "DataSocket Reference"={"CWDSLib._DCWDataSocket"=refnum, "CWDSLib._DCWData"=refnum, "OnDataUpdated"=0, "OnStatusUpdated"=0}}, "AT at vent ATS Home pos"={"Tag Name"="S060.PXI.Signals.PlltData.SN", "Network Path"="172.15.51.1,1,0", "use opc"=FALSE, "DataSocket Reference"={"CWDSLib._DCWDataSocket"=refnum, "CWDSLib._DCWData"=refnum, "OnDataUpdated"=0, "OnStatusUpdated"=0}}, "Start Adjust LVDT"={"Tag Name"="S060.PXI.Signals.PlltData.SN", "Network Path"="172.15.51.1,1,0", "use opc"=FALSE, "DataSocket Reference"={"CWDSLib._DCWDataSocket"=refnum, "CWDSLib._DCWData"=refnum, "OnDataUpdated"=0, "OnStatusUpdated"=0}}, "Finish Adjust LVDT"={"Tag Name"="S060.PXI.Signals.PlltData.SN", "Network Path"="172.15.51.1,1,0", "use opc"=FALSE, "DataSocket Reference"={"CWDSLib._DCWDataSocket"=refnum, "CWDSLib._DCWData"=refnum, "OnDataUpdated"=0, "OnStatusUpdated"=0}}} {"AT in sunshad wand up pos"."DataSocket Reference"."OnStatusUpdated" format="%.0x"; "AT in sunshad wand up pos"."DataSocket Reference"."OnDataUpdated" format="%.0x"; "AT in glass wand up pos"."DataSocket Reference"."OnStatusUpdated" format="%.0x"; "AT in glass wand up pos"."DataSocket Reference"."OnDataUpdated" format="%.0x"; "Finish Adjust LVDT"."DataSocket Reference"."OnStatusUpdated" format="%.0x"; "Finish Adjust LVDT"."DataSocket Reference"."OnDataUpdated" format="%.0x"; "Start Adjust LVDT"."DataSocket Reference"."OnStatusUpdated" format="%.0x"; "Start Adjust LVDT"."DataSocket Reference"."OnDataUpdated" format="%.0x"; "AT at vent ATS Home pos"."DataSocket Reference"."OnStatusUpdated" format="%.0x"; "AT at vent ATS Home pos"."DataSocket Reference"."OnDataUpdated" format="%.0x"; "AT at vent ATS test pos"."DataSocket Reference"."OnStatusUpdated" format="%.0x"; "AT at vent ATS test pos"."DataSocket Reference"."OnDataUpdated" format="%.0x"; "NVH Operator Re-do"."DataSocket Reference"."OnStatusUpdated" format="%.0x"; "NVH Operator Re-do"."DataSocket Reference"."OnDataUpdated" format="%.0x"; "NVH Operator Express Glass Vent Close"."DataSocket Reference"."OnStatusUpdated" format="%.0x"; "NVH Operator Express Glass Vent Close"."DataSocket Reference"."OnDataUpdated" format="%.0x"; "NVH Operator Express Glass vent Open"."DataSocket Reference"."OnStatusUpdated" format="%.0x"; "NVH Operator Express Glass vent Open"."DataSocket Reference"."OnDataUpdated" format="%.0x"; "windproof position"."DataSocket Reference"."OnStatusUpdated" format="%.0x"; "windproof position"."DataSocket Reference"."OnDataUpdated" format="%.0x"; "NVH Operator Check"."DataSocket Reference"."OnStatusUpdated" format="%.0x"; "NVH Operator Check"."DataSocket Reference"."OnDataUpdated" format="%.0x"; "NVH Operator Finish"."DataSocket Reference"."OnStatusUpdated" format="%.0x"; "NVH Operator Finish"."DataSocket Reference"."OnDataUpdated" format="%.0x"; "NVH Operator Glass Close Noise"."DataSocket Reference"."OnStatusUpdated" format="%.0x"; "NVH Operator Glass Close Noise"."DataSocket Reference"."OnDataUpdated" format="%.0x"; "NVH Operator Glass Open Noise"."DataSocket Reference"."OnStatusUpdated" format="%.0x"; "NVH Operator Glass Open Noise"."DataSocket Reference"."OnDataUpdated" format="%.0x"; "NVH Operator Sunshade Close Noise"."DataSocket Reference"."OnStatusUpdated" format="%.0x"; "NVH Operator Sunshade Close Noise"."DataSocket Reference"."OnDataUpdated" format="%.0x"; "NVH Operator Sunshade Open Noise"."DataSocket Reference"."OnStatusUpdated" format="%.0x"; "NVH Operator Sunshade Open Noise"."DataSocket Reference"."OnDataUpdated" format="%.0x"; "NVH Operator Vent Close Noise"."DataSocket Reference"."OnStatusUpdated" format="%.0x"; "NVH Operator Vent Close Noise"."DataSocket Reference"."OnDataUpdated" format="%.0x"; "NVH Operator Vent Open Noise"."DataSocket Reference"."OnStatusUpdated" format="%.0x"; "NVH Operator Vent Open Noise"."DataSocket Reference"."OnDataUpdated" format="%.0x"; "NVH Operator Express Rollo Close02"."DataSocket Reference"."OnStatusUpdated" format="%.0x"; "NVH Operator Express Rollo Close02"."DataSocket Reference"."OnDataUpdated" format="%.0x"; "NVH Operator Express Rollo Open02"."DataSocket Reference"."OnStatusUpdated" format="%.0x"; "NVH Operator Express Rollo Open02"."DataSocket Reference"."OnDataUpdated" format="%.0x"; "NVH Operator Express Rollo Close01"."DataSocket Reference"."OnStatusUpdated" format="%.0x"; "NVH Operator Express Rollo Close01"."DataSocket Reference"."OnDataUpdated" format="%.0x"; "NVH Operator Express Rollo Open01"."DataSocket Reference"."OnStatusUpdated" format="%.0x"; "NVH Operator Express Rollo Open01"."DataSocket Reference"."OnDataUpdated" format="%.0x"; "NVH Operator Express Glass Close"."DataSocket Reference"."OnStatusUpdated" format="%.0x"; "NVH Operator Express Glass Close"."DataSocket Reference"."OnDataUpdated" format="%.0x"; "NVH Operator Express Glass Open"."DataSocket Reference"."OnStatusUpdated" format="%.0x"; "NVH Operator Express Glass Open"."DataSocket Reference"."OnDataUpdated" format="%.0x"; "NVH Operator Fail"."DataSocket Reference"."OnStatusUpdated" format="%.0x"; "NVH Operator Fail"."DataSocket Reference"."OnDataUpdated" format="%.0x"; "NVH Operator Pass"."DataSocket Reference"."OnStatusUpdated" format="%.0x"; "NVH Operator Pass"."DataSocket Reference"."OnDataUpdated" format="%.0x"; "Z LVDTs Extended"."DataSocket Reference"."OnStatusUpdated" format="%.0x"; "Z LVDTs Extended"."DataSocket Reference"."OnDataUpdated" format="%.0x"; "Check Frame Barcode"."DataSocket Reference"."OnStatusUpdated" format="%.0x"; "Check Frame Barcode"."DataSocket Reference"."OnDataUpdated" format="%.0x"; "SS Barcode Scanner Bypassed"."DataSocket Reference"."OnStatusUpdated" format="%.0x"; "SS Barcode Scanner Bypassed"."DataSocket Reference"."OnDataUpdated" format="%.0x"; "AT VentPMACisExtend"."DataSocket Reference"."OnStatusUpdated" format="%.0x"; "AT VentPMACisExtend"."DataSocket Reference"."OnDataUpdated" format="%.0x"; "AT VentPMACatHome"."DataSocket Reference"."OnStatusUpdated" format="%.0x"; "AT VentPMACatHome"."DataSocket Reference"."OnDataUpdated" format="%.0x"; "wind deflector low speed pos"."DataSocket Reference"."OnStatusUpdated" format="%.0x"; "wind deflector low speed pos"."DataSocket Reference"."OnDataUpdated" format="%.0x"; "wind deflector high speed pos"."DataSocket Reference"."OnStatusUpdated" format="%.0x"; "wind deflector high speed pos"."DataSocket Reference"."OnDataUpdated" format="%.0x"; "control slide right over stroke"."DataSocket Reference"."OnStatusUpdated" format="%.0x"; "control slide right over stroke"."DataSocket Reference"."OnDataUpdated" format="%.0x"; "control slide right good"."DataSocket Reference"."OnStatusUpdated" format="%.0x"; "control slide right good"."DataSocket Reference"."OnDataUpdated" format="%.0x"; "control slide left over stroke"."DataSocket Reference"."OnStatusUpdated" format="%.0x"; "control slide left over stroke"."DataSocket Reference"."OnDataUpdated" format="%.0x"; "control slide left good"."DataSocket Reference"."OnStatusUpdated" format="%.0x"; "control slide left good"."DataSocket Reference"."OnDataUpdated" format="%.0x"; "control slide at home"."DataSocket Reference"."OnStatusUpdated" format="%.0x"; "control slide at home"."DataSocket Reference"."OnDataUpdated" format="%.0x"; "ss servo closing"."DataSocket Reference"."OnStatusUpdated" format="%.0x"; "ss servo closing"."DataSocket Reference"."OnDataUpdated" format="%.0x"; "ss servo opening"."DataSocket Reference"."OnStatusUpdated" format="%.0x"; "ss servo opening"."DataSocket Reference"."OnDataUpdated" format="%.0x"; "ss servo at close"."DataSocket Reference"."OnStatusUpdated" format="%.0x"; "ss servo at close"."DataSocket Reference"."OnDataUpdated" format="%.0x"; "ss servo at open"."DataSocket Reference"."OnStatusUpdated" format="%.0x"; "ss servo at open"."DataSocket Reference"."OnDataUpdated" format="%.0x"; "manual barcode print"."DataSocket Reference"."OnStatusUpdated" format="%.0x"; "manual barcode print"."DataSocket Reference"."OnDataUpdated" format="%.0x"; "LVDT's Retracted"."DataSocket Reference"."OnStatusUpdated" format="%.0x"; "LVDT's Retracted"."DataSocket Reference"."OnDataUpdated" format="%.0x"; "abort"."DataSocket Reference"."OnStatusUpdated" format="%.0x"; "abort"."DataSocket Reference"."OnDataUpdated" format="%.0x"; "start"."DataSocket Reference"."OnStatusUpdated" format="%.0x"; "start"."DataSocket Reference"."OnDataUpdated" format="%.0x"; "bolt check 8"."DataSocket Reference"."OnStatusUpdated" format="%.0x"; "bolt check 8"."DataSocket Reference"."OnDataUpdated" format="%.0x"; "bolt check 7"."DataSocket Reference"."OnStatusUpdated" format="%.0x"; "bolt check 7"."DataSocket Reference"."OnDataUpdated" format="%.0x"; "bolt check 6"."DataSocket Reference"."OnStatusUpdated" format="%.0x"; "bolt check 6"."DataSocket Reference"."OnDataUpdated" format="%.0x"; "bolt check 5"."DataSocket Reference"."OnStatusUpdated" format="%.0x"; "bolt check 5"."DataSocket Reference"."OnDataUpdated" format="%.0x"; "bolt check 4"."DataSocket Reference"."OnStatusUpdated" format="%.0x"; "bolt check 4"."DataSocket Reference"."OnDataUpdated" format="%.0x"; "bolt check 3"."DataSocket Reference"."OnStatusUpdated" format="%.0x"; "bolt check 3"."DataSocket Reference"."OnDataUpdated" format="%.0x"; "bolt check 2"."DataSocket Reference"."OnStatusUpdated" format="%.0x"; "bolt check 2"."DataSocket Reference"."OnDataUpdated" format="%.0x"; "bolt check 1"."DataSocket Reference"."OnStatusUpdated" format="%.0x"; "bolt check 1"."DataSocket Reference"."OnDataUpdated" format="%.0x"; "LVDT's Extended"."DataSocket Reference"."OnStatusUpdated" format="%.0x"; "LVDT's Extended"."DataSocket Reference"."OnDataUpdated" format="%.0x"; "AT in wand home pos"."DataSocket Reference"."OnStatusUpdated" format="%.0x"; "AT in wand home pos"."DataSocket Reference"."OnDataUpdated" format="%.0x"; "AT in sunshad wand lower pos"."DataSocket Reference"."OnStatusUpdated" format="%.0x"; "AT in sunshad wand lower pos"."DataSocket Reference"."OnDataUpdated" format="%.0x"; "AT in glass wand lower pos"."DataSocket Reference"."OnStatusUpdated" format="%.0x"; "AT in glass wand lower pos"."DataSocket Reference"."OnDataUpdated" format="%.0x"; "AT shade position"."DataSocket Reference"."OnStatusUpdated" format="%.0x"; "AT shade position"."DataSocket Reference"."OnDataUpdated" format="%.0x"; "AT glass position"."DataSocket Reference"."OnStatusUpdated" format="%.0x"; "AT glass position"."DataSocket Reference"."OnDataUpdated" format="%.0x"}) -> (0 "Operator Finish?":bool, 1 "Noise Source output":u32, 3 "Error Table Out":string[][](table))   [LabVIEW 2018]
uses:
  02.Type Def's/station plc read boolean tags.ctl
  05.UserVI's/type defs/plc path and tag.ctl
  <vilib>/Platform/dataskt.llb/DataSocket Reference Type.ctl
  02.Type Def's/station plc write boolean tags.ctl
panel:
  # "start/abort only used by barcode instance, since there are discrete signals for this in the other stations."
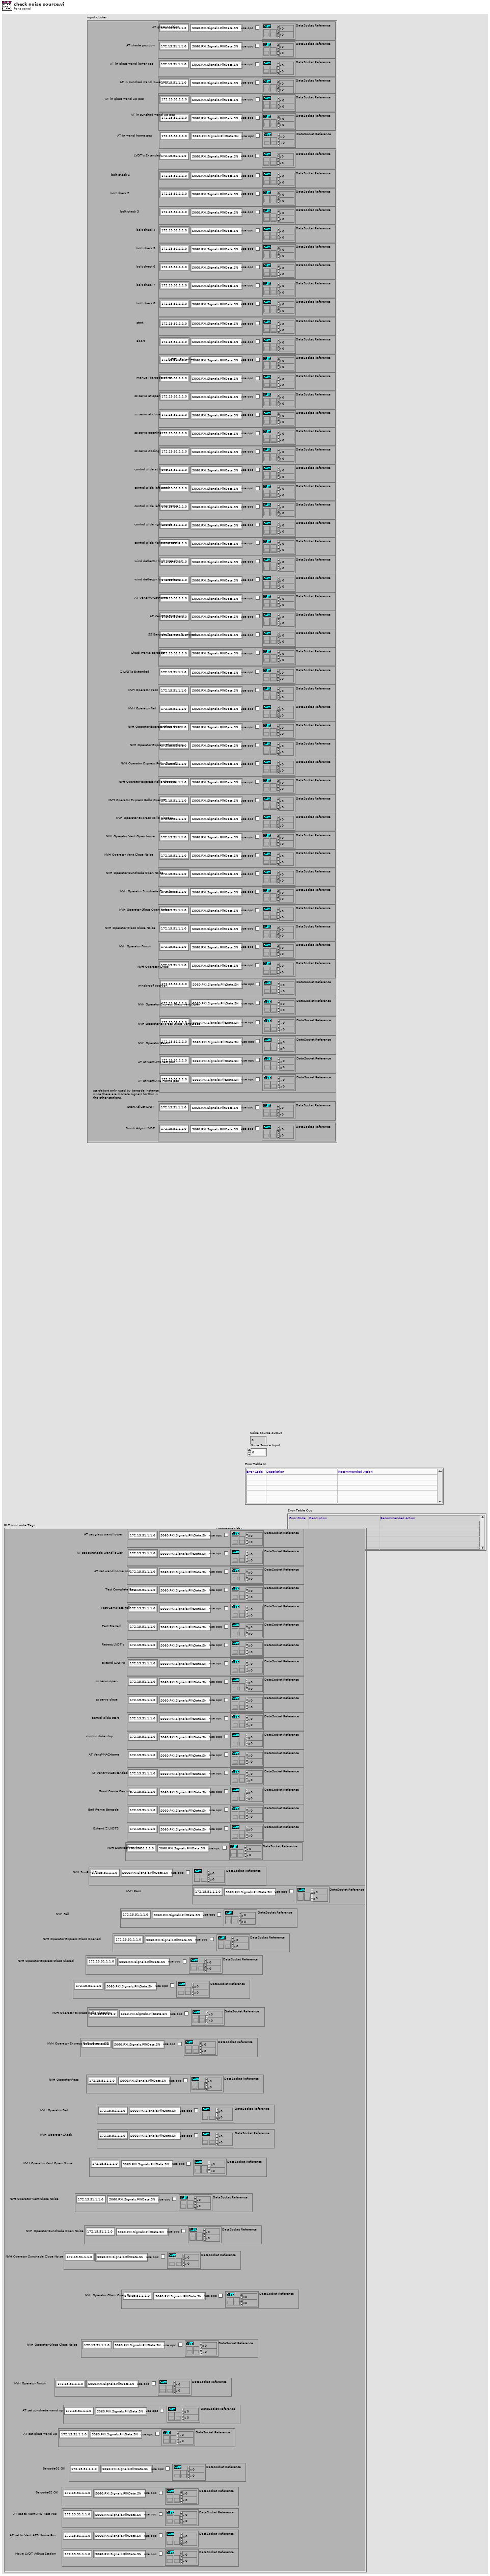
[diagram p1: front panel]
types:
  T1 = typedef "station plc write boolean tags.ctl" = cluster{"AT set glass wand lower":T2, "AT set sunshade wand lower":T2, "AT set sunshade wand up":T2, "AT set glass wand up":T2, "AT set wand home pos":T2, "Test Complete Pass":T2, "Test Complete Fail":T2, "Test Started":T2, "Retract LVDT's":T2, "Extend LVDT's":T2, "ss servo open":T2, "ss servo close":T2, "control slide start":T2, "control slide stop":T2, "AT VentPMACHome":T2, "AT VentPMACExtended":T2, "Good Frame Barcode":T2, "Bad Frame Barcode":T2, "Extend Z LVDTS":T2, "NVH SunRoof Moving":T2, "NVH SunRoof Stop":T2, "NVH Pass":T2, "NVH Fail":T2, "NVH Operator Express Glass Opened":T2, "NVH Operator Express Glass Closed":T2, "NVH Operator Express Rollo Opened01":T2, "NVH Operator Express Rollo Closed01":T2, "NVH Operator Express Rollo Opened02":T2, "NVH Operator Pass":T2, "NVH Operator Fail":T2, "NVH Operator Check":T2, "NVH Operator Vent Open Noise":T2, "NVH Operator Vent Close Noise":T2, "NVH Operator Sunshade Open Noise":T2, "NVH Operator Sunshade Close Noise":T2, "NVH Operator Glass Open Noise":T2, "NVH Operator Glass Close Noise":T2, "NVH Operator Finish":T2, "Barcode01 OK":T2, "Barcode02 OK":T2, "AT set to Vent ATS Test Pos":T2, "AT set to Vent ATS Home Pos":T2, "Move LVDT Adjust Station":T2}
  T2 = typedef "plc path and tag.ctl" = cluster{"Tag Name":string, "Network Path":string, "use opc":bool, "DataSocket Reference":T3}
  T3 = typedef "DataSocket Reference Type.ctl" = cluster{"CWDSLib._DCWDataSocket":refnum<k7>, "CWDSLib._DCWData":refnum<k7>, "OnDataUpdated":u32, "OnStatusUpdated":u32}
  T4 = typedef "station plc read boolean tags.ctl" = cluster{"AT glass position":T2, "AT shade position":T2, "AT in glass wand lower pos":T2, "AT in glass wand up pos":T2, "AT in sunshad wand lower pos":T2, "AT in sunshad wand up pos":T2, "AT in wand home pos":T2, "LVDT's Extended":T2, "bolt check 1":T2, "bolt check 2":T2, "bolt check 3":T2, "bolt check 4":T2, "bolt check 5":T2, "bolt check 6":T2, "bolt check 7":T2, "bolt check 8":T2, "start":T2, "abort":T2, "LVDT's Retracted":T2, "manual barcode print":T2, "ss servo at open":T2, "ss servo at close":T2, "ss servo opening":T2, "ss servo closing":T2, "control slide at home":T2, "control slide left good":T2, "control slide left over stroke":T2, "control slide right good":T2, "control slide right over stroke":T2, "wind deflector high speed pos":T2, "wind deflector low speed pos":T2, "AT VentPMACatHome":T2, "AT VentPMACisExtend":T2, "SS Barcode Scanner Bypassed":T2, "Check Frame Barcode":T2, "Z LVDTs Extended":T2, "NVH Operator Pass":T2, "NVH Operator Fail":T2, "NVH Operator Express Glass Open":T2, "NVH Operator Express Glass Close":T2, "NVH Operator Express Rollo Open01":T2, "NVH Operator Express Rollo Close01":T2, "NVH Operator Express Rollo Open02":T2, "NVH Operator Express Rollo Close02":T2, "NVH Operator Vent Open Noise":T2, "NVH Operator Vent Close Noise":T2, "NVH Operator Sunshade Open Noise":T2, "NVH Operator Sunshade Close Noise":T2, "NVH Operator Glass Open Noise":T2, "NVH Operator Glass Close Noise":T2, "NVH Operator Finish":T2, "NVH Operator Check":T2, "windproof position":T2, "NVH Operator Express Glass vent Open":T2, "NVH Operator Express Glass Vent Close":T2, "NVH Operator Re-do":T2, "AT at vent ATS test pos":T2, "AT at vent ATS Home pos":T2, "Start Adjust LVDT":T2, "Finish Adjust LVDT":T2}
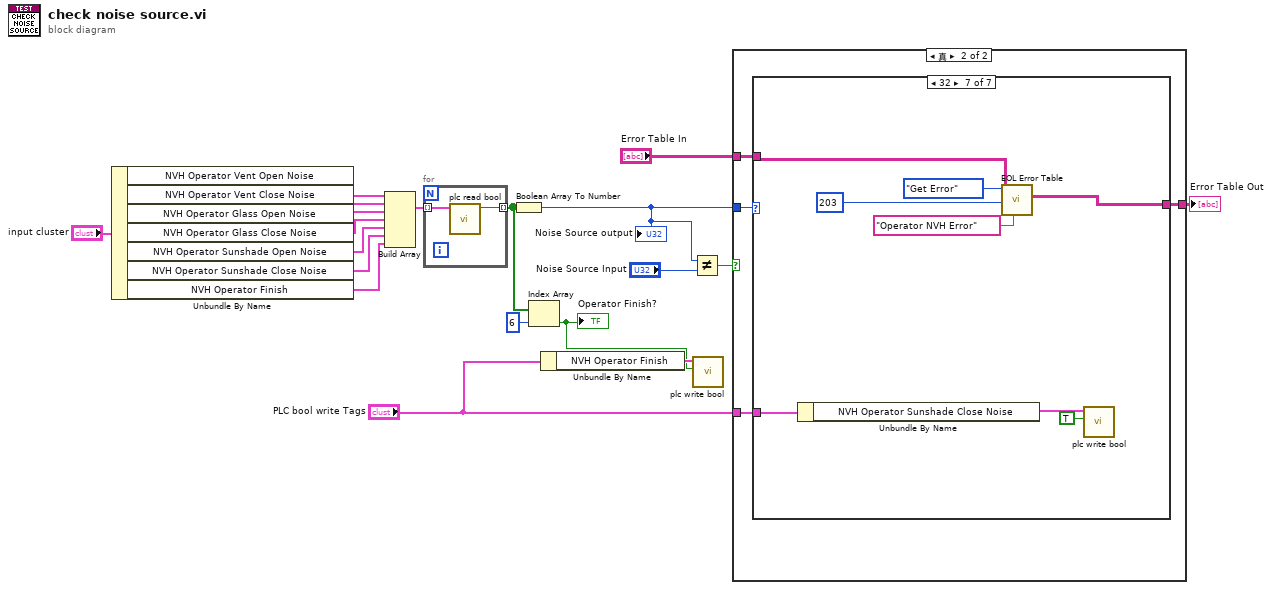
[diagram p0: block diagram]
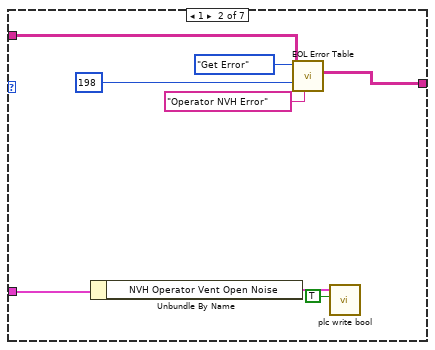
[diagram p4: hidden frame]
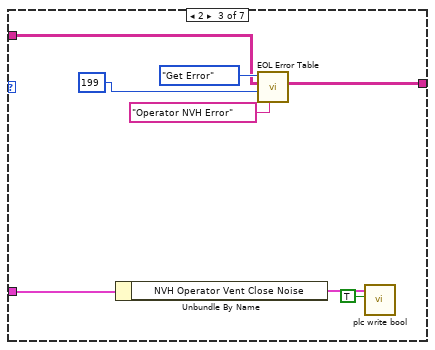
[diagram p5: hidden frame]
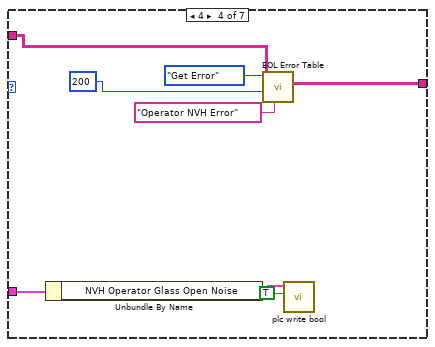
[diagram p6: hidden frame]
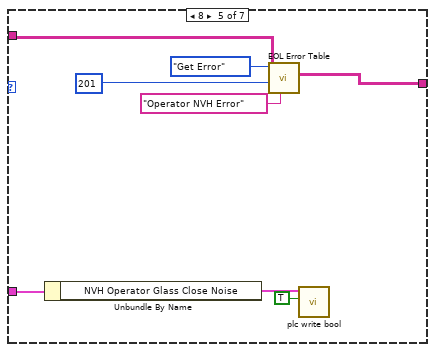
[diagram p7: hidden frame]
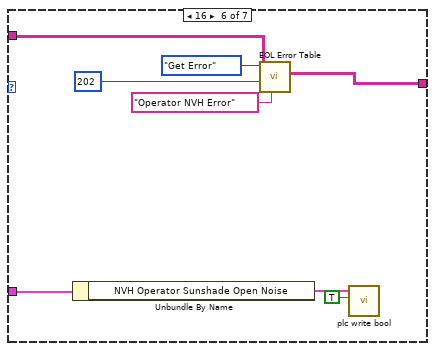
[diagram p8: hidden frame]
diagram:
  n1 = Unbundle By Name("input cluster") -> ("NVH Operator Vent Open Noise"=w18:T2, "NVH Operator Vent Close Noise"=w17:T2, "NVH Operator Glass Open Noise"=w16:T2, "NVH Operator Glass Close Noise"=w15:T2, "NVH Operator Sunshade Open Noise"=w14:T2, "NVH Operator Sunshade Close Noise"=w13:T2, "NVH Operator Finish"=w12:T2)
  n2 = Build Array(w18, w17, w16, w15, w14, w13, w12) -> (w11:T2[])
  n3 = for {
    tunnel: w11 -> [w21] mode=indexing
    tunnel: [w20] -> w9 mode=indexing
    n4 = call "plc read bool.vi"("addr,tag"=w21) -> ("value"=w20:bool)  [unwired: 9 in, 1 out]
  }
  n5 = Boolean Array To Number(Boolean array=w9) -> (number=w6:u32)
  "Noise Source output" <- w6
  n6 = Index Array(array=w9, index=6) -> (element=w1:bool)
  "Operator Finish?" <- w1
  n7 = Unbundle By Name("PLC bool write Tags") -> ("NVH Operator Finish"=w3:T2)
  n8 = Not Equal?(x=w6, y="Noise Source Input") -> (x != y?=w4:bool)
  n9 = call "plc write bool.vi"("value"=w1, "addr,tag"=w3) -> ()  [unwired: 9 in, 1 out]
  n10 = case shown="真" w4 {
    tunnel: "Error Table In" -> [w22 w26]
    tunnel: [w22 w25] -> w7
    tunnel: w6 -> [_ w24]
    tunnel: "PLC bool write Tags" -> [_ w23]
    frame False {
    }
    frame True {
      n11 = case shown="32" w24 {
        tunnel: w26 -> [w27 w32 w40 w48 w56 w64 w72]
        tunnel: [w27 w31 w39 w47 w55 w63 w71] -> w25
        tunnel: w23 -> [_ w30 w38 w45 w54 w62 w70]
        frame 0, Default {
        }
        frame 1 {
          n12 = Unbundle By Name(w30) -> ("NVH Operator Vent Open Noise"=w29:T2)
          n13 = call "EOL Error Table.vi"("Error Description"="Operator NVH Error", "Error No."=u16 198, "Error Table In"=w32, "Error Mode"=enum16{"Init", "Get Error"}."Get Error") -> ("Error Table Out"=w31:string[][])  [unwired: 6 in, 1 out]
          n14 = call "plc write bool.vi"("value"=TRUE, "addr,tag"=w29) -> ()  [unwired: 9 in, 1 out]
        }
        frame 2 {
          n15 = Unbundle By Name(w38) -> ("NVH Operator Vent Close Noise"=w37:T2)
          n16 = call "EOL Error Table.vi"("Error Description"="Operator NVH Error", "Error No."=u16 199, "Error Table In"=w40, "Error Mode"=enum16{"Init", "Get Error"}."Get Error") -> ("Error Table Out"=w39:string[][])  [unwired: 6 in, 1 out]
          n17 = call "plc write bool.vi"("value"=TRUE, "addr,tag"=w37) -> ()  [unwired: 9 in, 1 out]
        }
        frame 4 {
          n18 = Unbundle By Name(w45) -> ("NVH Operator Glass Open Noise"=w46:T2)
          n19 = call "EOL Error Table.vi"("Error Description"="Operator NVH Error", "Error No."=u16 200, "Error Table In"=w48, "Error Mode"=enum16{"Init", "Get Error"}."Get Error") -> ("Error Table Out"=w47:string[][])  [unwired: 6 in, 1 out]
          n20 = call "plc write bool.vi"("value"=TRUE, "addr,tag"=w46) -> ()  [unwired: 9 in, 1 out]
        }
        frame 8 {
          n21 = Unbundle By Name(w54) -> ("NVH Operator Glass Close Noise"=w53:T2)
          n22 = call "EOL Error Table.vi"("Error Description"="Operator NVH Error", "Error No."=u16 201, "Error Table In"=w56, "Error Mode"=enum16{"Init", "Get Error"}."Get Error") -> ("Error Table Out"=w55:string[][])  [unwired: 6 in, 1 out]
          n23 = call "plc write bool.vi"("value"=TRUE, "addr,tag"=w53) -> ()  [unwired: 9 in, 1 out]
        }
        frame 16 {
          n24 = Unbundle By Name(w62) -> ("NVH Operator Sunshade Open Noise"=w61:T2)
          n25 = call "EOL Error Table.vi"("Error Description"="Operator NVH Error", "Error No."=u16 202, "Error Table In"=w64, "Error Mode"=enum16{"Init", "Get Error"}."Get Error") -> ("Error Table Out"=w63:string[][])  [unwired: 6 in, 1 out]
          n26 = call "plc write bool.vi"("value"=TRUE, "addr,tag"=w61) -> ()  [unwired: 9 in, 1 out]
        }
        frame 32 {
          n27 = Unbundle By Name(w70) -> ("NVH Operator Sunshade Close Noise"=w69:T2)
          n28 = call "EOL Error Table.vi"("Error Description"="Operator NVH Error", "Error No."=u16 203, "Error Table In"=w72, "Error Mode"=enum16{"Init", "Get Error"}."Get Error") -> ("Error Table Out"=w71:string[][])  [unwired: 6 in, 1 out]
          n29 = call "plc write bool.vi"("value"=TRUE, "addr,tag"=w69) -> ()  [unwired: 9 in, 1 out]
        }
      }
    }
  }
  "Error Table Out" <- w7
